vi "Get Table.vi"(7 "Update Method (New Top)":T1=enum."New Top", 11 "Cyclic Table in":refnum<class "Cyclic Table.lvclass">) -> (2 "Table Data (sorted by time)":string[][](array[string]))   [LabVIEW 2024, in "Cyclic Table.lvclass"]
doc: "Get the current table array."
uses:
  Cyclic Table.lvclass
  Cyclic Table.lvclass/Cyclic Table.ctl
  Update Method.ctl
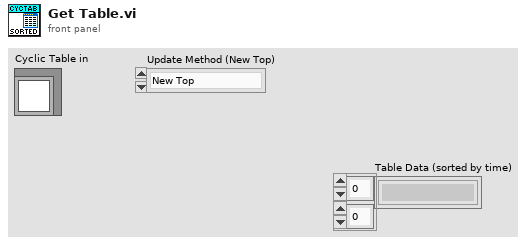
[diagram p1: front panel]
types:
  T1 = typedef "Cyclic Table.lvclass/Update Method.ctl" = enum16{"Cyclic", "Old Top", "New Top"}
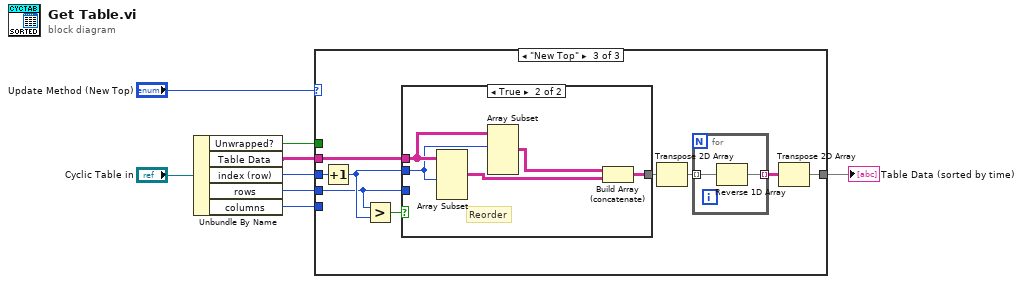
[diagram p0: block diagram]
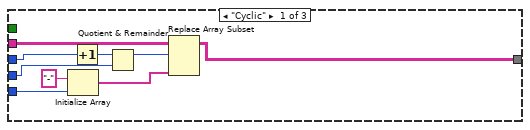
[diagram p2: hidden frame]
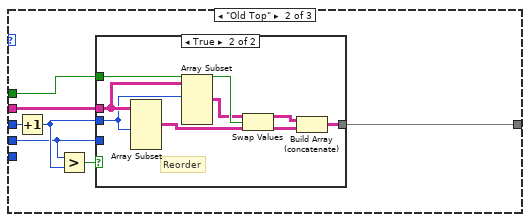
[diagram p3: hidden frame]
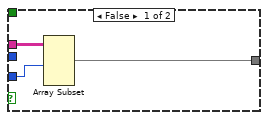
[diagram p4: hidden frame]
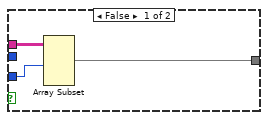
[diagram p5: hidden frame]
diagram:
  n1 = Unbundle By Name("Cyclic Table in") -> ("Unwrapped?"=w3:bool, "Table Data"=w7:string[][], "index (row)"=w5:i32, "rows"=w4:i32, "columns"=w2:i32)
  n2 = case shown="\"New Top\"" "Update Method (New Top)" {
    tunnel: w5 -> [w13 w22 w42]
    tunnel: w4 -> [w9 w21 w41]
    tunnel: w7 -> [w17 w20 w40]
    tunnel: [w11 w19 w36] -> w6
    tunnel: w3 -> [_ w18 _]
    tunnel: w2 -> [w15 _ _]
    frame "Cyclic" {
      n3 = Initialize Array("-", w15) -> (w14:string[])
      n4 = Increment(x=w13) -> (x+1=w12:i32)
      n5 = Quotient & Remainder(x=w12, y=w9) -> (x-y*floor(x/y)=w10:i32)  [unwired: 1 out]
      n6 = Replace Array Subset(array=w17, new element=w14, index (row)=w10) -> (w11:string[][])  [unwired: 1 in]
    }
    frame "Old Top" {
      n7 = Increment(x=w22) -> (x+1=w23:i32)
      n8 = Greater?(x=w21, y=w23) -> (0:w24:bool)
      n9 = case shown="True" w24 {
        tunnel: w20 -> [w27 w34]
        tunnel: [w26 w35] -> w19
        tunnel: w21 -> [w25 _]
        tunnel: w23 -> [_ w33]
        tunnel: w18 -> [_ w32]
        frame False {
          n10 = Array Subset(array=w27, length (row)=w25) -> (w26:string[][])  [unwired: 3 in]
        }
        frame True {
          # "Reorder"
          n11 = Array Subset(array=w34, length (row)=w33) -> (w30:string[][])  [unwired: 3 in]
          n12 = Array Subset(array=w34, index (row)=w33) -> (w31:string[][])  [unwired: 3 in]
          n13 = Swap Values(12:w31, 13:w32, 14:w30) -> (1:w28:string[][], 3:w29:string[][])
          n14 = Build Array (concatenate)(w28, w29) -> (w35:string[][])
        }
      }
    }
    frame "New Top" {
      n15 = Increment(x=w42) -> (x+1=w43:i32)
      n16 = Greater?(x=w41, y=w43) -> (0:w44:bool)
      n17 = case shown="True" w44 {
        tunnel: w40 -> [w49 w53]
        tunnel: [w48 w54] -> w39
        tunnel: w41 -> [w47 _]
        tunnel: w43 -> [_ w52]
        frame False {
          n18 = Array Subset(array=w49, length (row)=w47) -> (w48:string[][])  [unwired: 3 in]
        }
        frame True {
          # "Reorder"
          n19 = Array Subset(array=w53, length (row)=w52) -> (w51:string[][])  [unwired: 3 in]
          n20 = Array Subset(array=w53, index (row)=w52) -> (w50:string[][])  [unwired: 3 in]
          n21 = Build Array (concatenate)(w50, w51) -> (w54:string[][])
        }
      }
      n22 = Transpose 2D Array(2D array=w39) -> (transposed array=w38:string[][])
      n23 = for {
        tunnel: w38 -> [w46] mode=indexing
        tunnel: [w45] -> w37 mode=indexing
        n24 = Reverse 1D Array(array=w46) -> (reversed array=w45:string[])
      }
      n25 = Transpose 2D Array(2D array=w37) -> (transposed array=w36:string[][])
    }
  }
  "Table Data (sorted by time)" <- w6
